vi "Filter StrArray By Input.vi"(8 "Filter String":string, 11 "Array In":string[](array[string])) -> (3 "Array":string[](array[string]))   [LabVIEW 2017]
uses:
  Communicable State Machine.lvlib
  _Shared/CSM Shared.lvlib
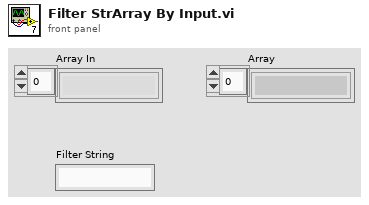
[diagram p1: front panel]
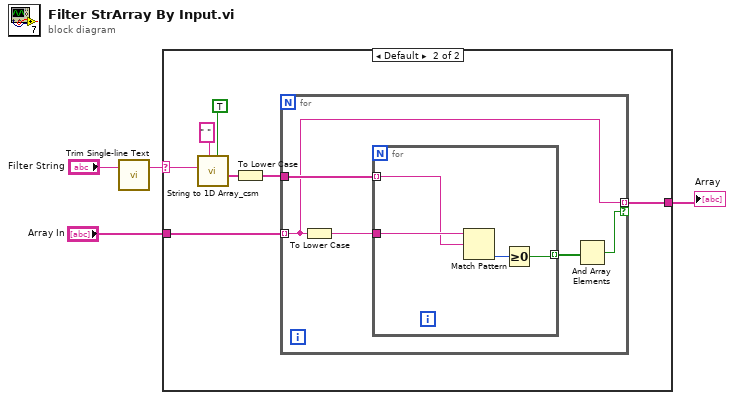
[diagram p0: block diagram]
diagram:
  n1 = call "Trim Single-line Text.vi"("single-line text"="Filter String") -> ("trimed text"=w1:string)  [unwired: 2 in]
  n2 = case shown="Default" w1 {
    selector: w1 -> [_ w6]
    tunnel: [w5 w12] -> w4
    tunnel: "Array In" -> [w5 w7]
    frame "False" {
    }
    frame Default {
      n3 = call "String to 1D Array_csm.vi"("ignore duplicate delimiters? (F=No)"=TRUE, "delimiter (Tab)"=" ", "string"=w6) -> ("Array of Strings"=w8:string[])  [unwired: 8 in]
      n4 = To Lower Case(string=w8) -> (all lower case string=w9:string[])
      n5 = for {
        tunnel: w7 -> [w15] mode=indexing
        tunnel: w9 -> [w16]
        tunnel: [w15] -> w12 mode=indexing if=w14
        n6 = To Lower Case(string=w15) -> (all lower case string=w17:string)
        n7 = for {
          tunnel: w17 -> [w21]
          tunnel: [w19] -> w13 mode=indexing
          tunnel: w16 -> [w18] mode=indexing
          n8 = Match Pattern(string=w21, regular expression=w18) -> (offset past match=w20:i32)  [unwired: 1 in, 3 out]
          n9 = Greater Or Equal To 0?(x=w20) -> (x >= 0?=w19:bool)
        }
        n10 = And Array Elements(Boolean array=w13) -> (logical AND=w14:bool)
      }
    }
  }
  "Array" <- w4
